vi "myRIO_BRig_RT_dataCurrent_Irewarded.vi"() -> (2 "output_I_rewarded":i32)   [LabVIEW 2014]
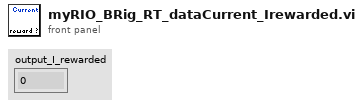
[diagram p1: front panel]
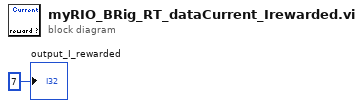
[diagram p0: block diagram]
diagram:
  "output_I_rewarded" <- 7 ("output_iBlock")
